vi "Sensor_Values.vi"() -> ()   [LabVIEW 2018]
panel:
  out "In_Motion":bool
  in  "Front_Climb_Velocity":dbl
  in  "Ball_IR":dbl
  out "In_Threshold":bool
  in  "Camera_Data":T1
  out "Climb_IR _Rear":bool
  out "Rezero":bool
  out "Climb_IR":bool
  in  "Back_Climb_Position":dbl
  out "Ball_Intaken":bool
  in  "Elevator_Position":dbl
  in  "Joint_Position":dbl
  out "Bottom_Joint_Limit":bool
  out "Top_Joint_Limit":bool
  out "Bottom_Elevator_Limit":bool
  out "Top_Elevator_Limit":bool
  out "Bottom_Climb_Limit_Front":bool
  out "Top_Climb_Limit_Front":bool
  out "Bottom_Climb_Limit_Back":bool
  out "Top_Climb_Limit_Back":bool
  in  "Front_Right_Drive":dbl
  in  "Back_Right_Drive":dbl
  in  "Back_Left_Drive":dbl
  in  "Front_Left_Drive":dbl
  in  "Front_Right_Azimuth":dbl
  in  "Back_Right_Azimuth":dbl
  in  "Back_Left_Azimuth":dbl
  in  "Front_Left_Azimuth":dbl
  in  "Yaw":dbl
  out "Back_Left_Limit":bool
  out "Front_Left_Limit":bool
  out "Back_Right_Limit":bool
  out "Front_Right_Limit":bool
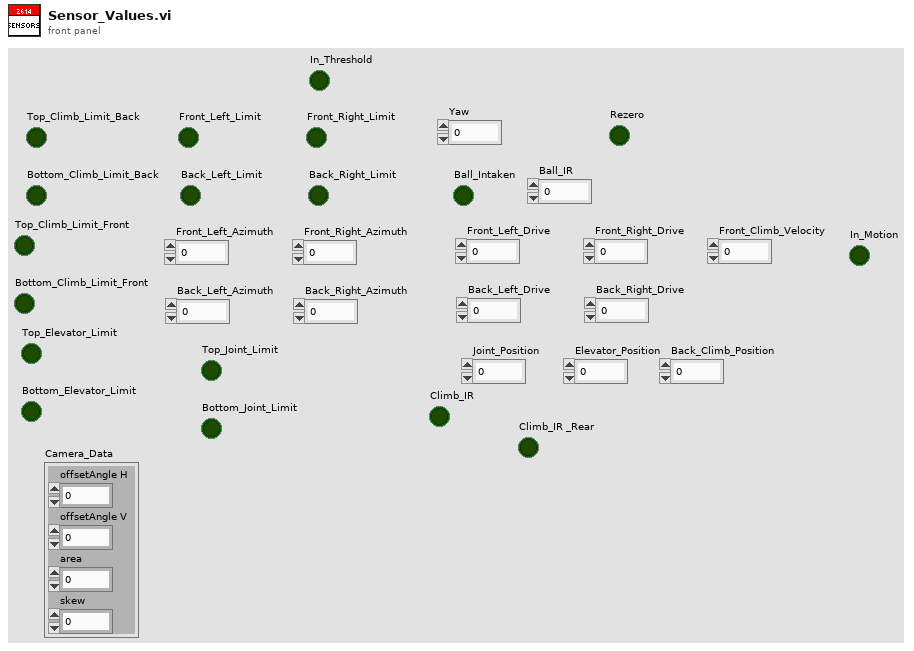
[diagram p1: front panel]
types:
  T1 = cluster{"offsetAngle H":dbl, "offsetAngle V":dbl, "area":dbl, "skew":dbl}
diagram:
